vi "RTM - Add Unbound Channels.vi"(8 "error in (no error)":errorcluster, 11 "Node Ptr":T1 format="%.0x") -> (0 "error out":errorcluster)   [LabVIEW 2019, in "UDP-Custom-Device System Explorer.lvlib"]
uses:
  UDP-Custom-Device System Explorer.lvlib
  <vilib>/NI VeriStand/Custom Device API/Custom Device Item Ref.ctl
  Shared/Types/Shared - Channel Data Type.ctl
  <vilib>/NI VeriStand/Custom Device API/Custom Device Channel.ctl
  <vilib>/NI VeriStand/Custom Device API/Custom Device Channel Type.ctl
  Shared/Constants.vi
  <vilib>/NI VeriStand/Custom Device API/Custom Device API.lvlib
  Shared/UDP-Custom-Device Shared.lvlib
  <vilib>/NI VeriStand/Custom Device Tools/Custom Device Utility Library/Custom Device Utility Library.lvlib
  Property Accessors/Rx Channel Accessors.lvlib
  Property Accessors/Rx Channel Section Accessors.lvlib
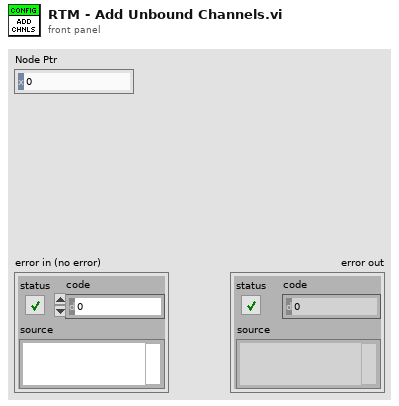
[diagram p1: front panel]
types:
  T1 = typedef "Custom Device API.lvlib/Custom Device Item Ref.ctl" = u64
  T2 = typedef "Custom Device API.lvlib/Custom Device Channel.ctl" = cluster{"Type":T3, "Units":string, "Default Value":dbl, "Faultable":bool, "Scalable":bool}
  T3 = typedef "Custom Device API.lvlib/Custom Device Channel Type.ctl" = enum16{"Input", "Output"}
  T4 = typedef "UDP-Custom-Device Shared.lvlib/Shared - Channel Data Type.ctl" = enum16{"Boolean", "Single", "Double", "I8", "I16", "I32", "I64", "U8", "U16", "U32", "U64"}
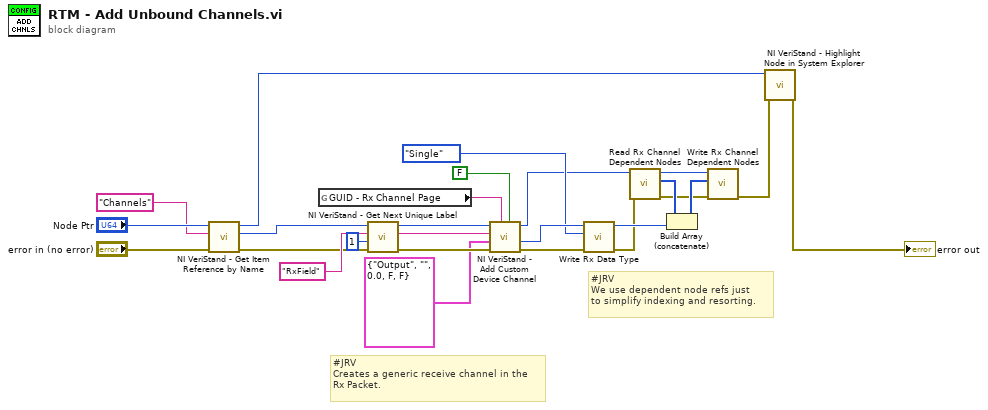
[diagram p0: block diagram]
diagram:
  # "#JRV\nWe use dependent node refs just\nto simplify indexing and resorting."
  # "#JRV\nCreates a generic receive channel in the \nRx Packet."
  n1 = call <vilib>:"NI VeriStand - Get Item Reference by Name.vi"("error in (no error)"="error in (no error)", "Item Name"="Channels" ("Section Name"), "Parent Ref in"="Node Ptr") -> ("error out"=w12:errorcluster, "Item Ref"=w11:T1, "Parent Ref out"=w10:T1)  [unwired: 5 in, 1 out]
  n2 = global read "Constants.vi" "GUID - Rx Channel Page"() -> (w26:string)
  n3 = call <vilib>:"NI VeriStand - Get Next Unique Label.vi"("error in (no error)"=w12, "Start Value (1)"=1, "Label"="RxField", "Parent Ref in"=w11) -> ("error out"=w23:errorcluster, "Label out"=w22:string, "Parent Ref dup"=w21:T1)  [unwired: 4 in, 1 out]
  n4 = call <vilib>:"NI VeriStand - Add Custom Device Channel.vi"("Highlight? (F)"=FALSE, "GUID (Default Channel)"=w26, "error in (no error)"=w23, "Channel"=T2 {"Type"=enum."Output", "Units"="", "Default Value"=0.0, "Faultable"=FALSE, "Scalable"=FALSE}, "Channel Name"=w22, "Parent Ref in"=w21) -> ("error out"=w18:errorcluster, "Channel Ref"=w19:T1, "Parent Ref out"=w7:T1)  [unwired: 2 in, 1 out]
  n5 = call "Write Rx Data Type.vi"("error in (no error)"=w18, "Data Type"=Shared_-_Channel_Data_Type."Single", "Node Ptr"=w19) -> ("error out"=w6:errorcluster, "Node Ptr out"=w9:T1)  [unwired: 7 in]
  n6 = call "Read Rx Channel Dependent Nodes.vi"("error in (no error)"=w6, "Node Ptr"=w7) -> ("error out"=w2:errorcluster, "Dependent Node Refs"=w4:T1[], "Node Ptr out"=w5:T1)  [unwired: 7 in]
  n7 = Build Array (concatenate)(w4, w9) -> (w3:T1[])
  n8 = call "Write Rx Channel Dependent Nodes.vi"("error in (no error)"=w2, "Dependent Node Refs"=w3, "Node Ptr"=w5) -> ("error out"=w1:errorcluster)  [unwired: 7 in, 1 out]
  n9 = call <vilib>:"NI VeriStand - Highlight Node in System Explorer.vi"("error in (no error)"=w1, "Item Ref in"=w10) -> ("error out"=→"error out":errorcluster)  [unwired: 8 in, 1 out]
